vi "array.vi"() -> ()   [LabVIEW 2015]
panel:
  out "Array 2":dbl[](array[numeric])
  out "Array":dbl[][](array[numeric])
  # "多為陣列，直接拉旁邊的縮放框框\n把東西再拖到Array裡面定義屬性"
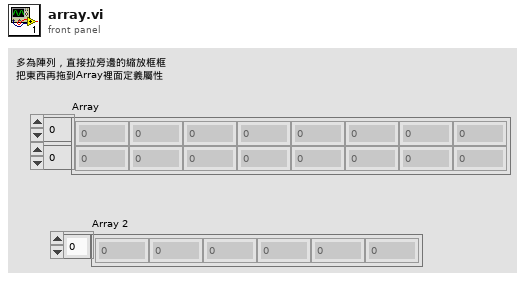
[diagram p1: front panel]
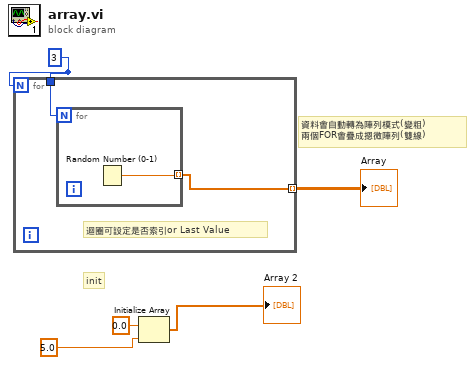
[diagram p0: block diagram]
diagram:
  w5 = 3
  # "init"
  # "資料會自動轉為陣列模式(變粗)\n兩個FOR會疊成摁微陣列(雙線)"
  n1 = for {
    N: w5 -> [_]
    tunnel: w5 -> [w7]
    tunnel: [w6] -> w4 mode=indexing
    # "迴圈可設定是否索引or Last Value"
    n2 = for {
      N: w7 -> [_]
      tunnel: [w8] -> w6 mode=indexing
      n3 = Random Number (0-1)() -> (number: 0 to 1=w8:dbl)
    }
  }
  "Array" <- w4
  n4 = Initialize Array(0.0 ("element"), 5.0 ("element")) -> (→"Array 2":dbl[])
